vi "save shape.vi"(8 "error in (no error)":errorcluster, 11 "BMC in":refnum<class "BMC.lvclass">) -> (0 "error out":errorcluster, 3 "BMC out":refnum<class "BMC.lvclass">)   [LabVIEW 2012, in "BMC.lvclass"]
uses:
  BMC.lvclass
  BMC.lvclass/BMC.ctl
  <vilib>/Utility/file.llb/Write To Spreadsheet File (DBL).vi
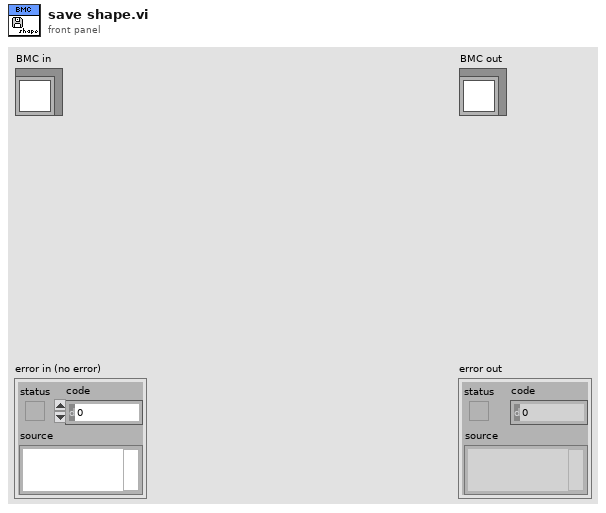
[diagram p1: front panel]
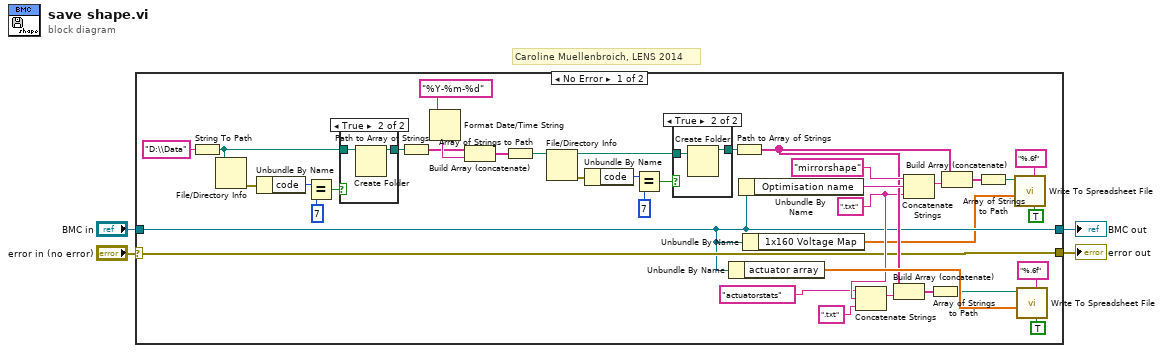
[diagram p0: block diagram]
diagram:
  # "Caroline Muellenbroich, LENS 2014"
  n1 = case shown="No Error" "error in (no error)" {
    selector: "error in (no error)" -> [w7 w50]
    tunnel: [w7 w50] -> w3
    tunnel: [w6 w49] -> w1
    tunnel: "BMC in" -> [w6 w49]
    frame No Error {
      w10 = ".txt" ("string")
      n2 = String To Path(string="D:\\Data") -> (path=w24:path)
      n3 = File/Directory Info(path=w24) -> (error out=w20:errorcluster)  [unwired: 1 in, 6 out]
      n4 = Unbundle By Name(w20) -> ("code"=w21:i32)
      n5 = Equal?(x=w21, y=7) -> (x = y?=w23:bool)
      n6 = case shown="True" w23 {
        tunnel: w24 -> [w46 w48]
        tunnel: [w46 w47] -> w26
        frame False {
        }
        frame True {
          n7 = Create Folder(path (use dialog)=w48) -> (created path=w47:path)  [unwired: 1 in, 3 out]
        }
      }
      n8 = Path to Array of Strings(0:w26) -> (2:w28:string[])  [unwired: 1 out]
      n9 = Format Date/Time String(time format string (%c)="%Y-%m-%d") -> (date/time string=w29:string)  [unwired: 2 out]
      n10 = Build Array (concatenate)(w28, w29) -> (w30:string[])
      n11 = Array of Strings to Path(0:w30) -> (2:w32:path)  [unwired: 1 out]
      n12 = File/Directory Info(path=w32) -> (path out=w36:path, error out=w33:errorcluster)  [unwired: 1 in, 5 out]
      n13 = Unbundle By Name(w33) -> ("code"=w34:i32)
      n14 = Equal?(x=w34, y=7) -> (x = y?=w35:bool)
      n15 = case shown="True" w35 {
        tunnel: w36 -> [w43 w45]
        tunnel: [w43 w44] -> w40
        frame False {
        }
        frame True {
          n16 = Create Folder(path (use dialog)=w45) -> (created path=w44:path)  [unwired: 1 in, 3 out]
        }
      }
      n17 = Unbundle By Name(w6) -> ("actuator array"=w15:dbl[])
      n18 = Path to Array of Strings(0:w40) -> (2:w11:string[])  [unwired: 1 out]
      n19 = Unbundle By Name(w6) -> ("Optimisation name"=w18:string)
      n20 = Unbundle By Name(w6) -> ("1x160 Voltage Map"=w5:dbl[])
      n21 = Concatenate Strings("actuatorstats" ("string"), w10, ".txt" ("string")) -> (w14:string)
      n22 = Build Array (concatenate)(w11, w14) -> (w13:string[])
      n23 = Concatenate Strings("mirrorshape" ("string"), w18, w10) -> (w37:string)
      n24 = Array of Strings to Path(0:w13) -> (2:w12:path)  [unwired: 1 in]
      n25 = Build Array (concatenate)(w11, w37) -> (w38:string[])
      n26 = Array of Strings to Path(0:w38) -> (2:w19:path)  [unwired: 1 in]
      n27 = call-poly <vilib>:"Write To Spreadsheet File.vi"("transpose? (no:F)"=TRUE, "format (%.3f)"="%.6f", "1D data"=w5, "file path (dialog if empty)"=w19) -> ()  [unwired: 2 in, 3 out]
      n28 = call-poly <vilib>:"Write To Spreadsheet File.vi"("transpose? (no:F)"=TRUE, "format (%.3f)"="%.6f", "1D data"=w15, "file path (dialog if empty)"=w12) -> ()  [unwired: 2 in, 3 out]
    }
    frame Error {
    }
  }
  "error out" <- w3
  "BMC out" <- w1
